vi "WIP_List.vi"(8 "error in (no error)":errorcluster, 10 "Label.Text":string, 11 "Ref in":T1={"MS SQL Connection"=refnum, "UDL File"=path "", "Time"="", "DCODE"="", "WIP+1"=0, "MC No?"=0, "POKAYOKE?"=FALSE, "Expected Result"="", "Result [Status]"="", "Clock"=0.0, "RFID"="", "WIP Queue"=refnum, "TS Parameter"={"ProfitCenterCode"="", "LineCode"="", "WorkOrderNumber"="", "Model"="", "Model_with_Prefix"="", "VendorCode"="", "SetParameterDateCode"="", "PokaYoke"=0, "Target"=1, "Live_DateCode"="", "CustomerPartNumber"="", "Hand"="", "sBarcode"=FALSE, "FCA"=0, "Ent_Stamp"=timestamp(0 s since 1904-01-01), "STS_CD"=0.0}, "Data_Queue"=[], "RFID Serial No."=""} {"TS Parameter"."FCA" format="%01d"; "TS Parameter"."Target" min=1 max=100000; "TS Parameter"."PokaYoke" min=0 max=1}) -> (0 "error out":errorcluster)   [LabVIEW 2020]
uses:
  Controls/TD SQL.ctl
  <vilib>/addons/database/Connection.llb/Conn ObjectReference.ctl
  Controls/WIP_State.ctl
  Controls/TS_Parameter.ctl
  MS SQL/MS_Global.vi
  <vilib>/addons/database/NI_Database_API.lvlib
panel:
  in  "Exit":bool
  in  "WIP List":i32(listbox)
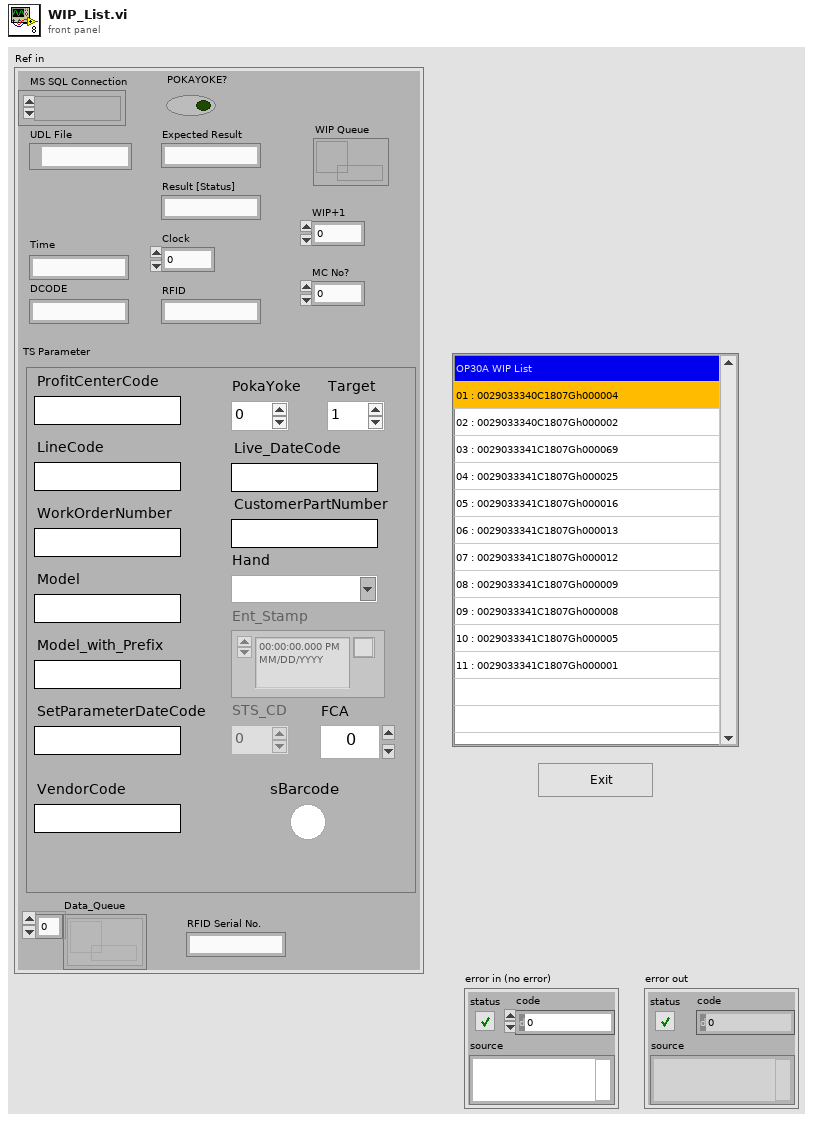
[diagram p1: front panel]
types:
  T1 = typedef "TD SQL.ctl" = cluster{"MS SQL Connection":T2, "UDL File":path, "Time":string, "DCODE":string, "WIP+1":i64, "MC No?":i32, "POKAYOKE?":bool, "Expected Result":string, "Result [Status]":string, "Clock":dbl, "RFID":string, "WIP Queue":refnum<queue>, "TS Parameter":T3, "Data_Queue":refnum<queue>[], "RFID Serial No.":string}
  T2 = typedef "NI_Database_API.lvlib/Conn ObjectReference.ctl" = refnum<k1>
  T3 = typedef "TS_Parameter.ctl" = cluster{"ProfitCenterCode":string, "LineCode":string, "WorkOrderNumber":string, "Model":string, "Model_with_Prefix":string, "VendorCode":string, "SetParameterDateCode":string, "PokaYoke":i32, "Target":i32, "Live_DateCode":string, "CustomerPartNumber":string, "Hand":string, "sBarcode":bool, "FCA":i32, "Ent_Stamp":timestamp, "STS_CD":dbl}
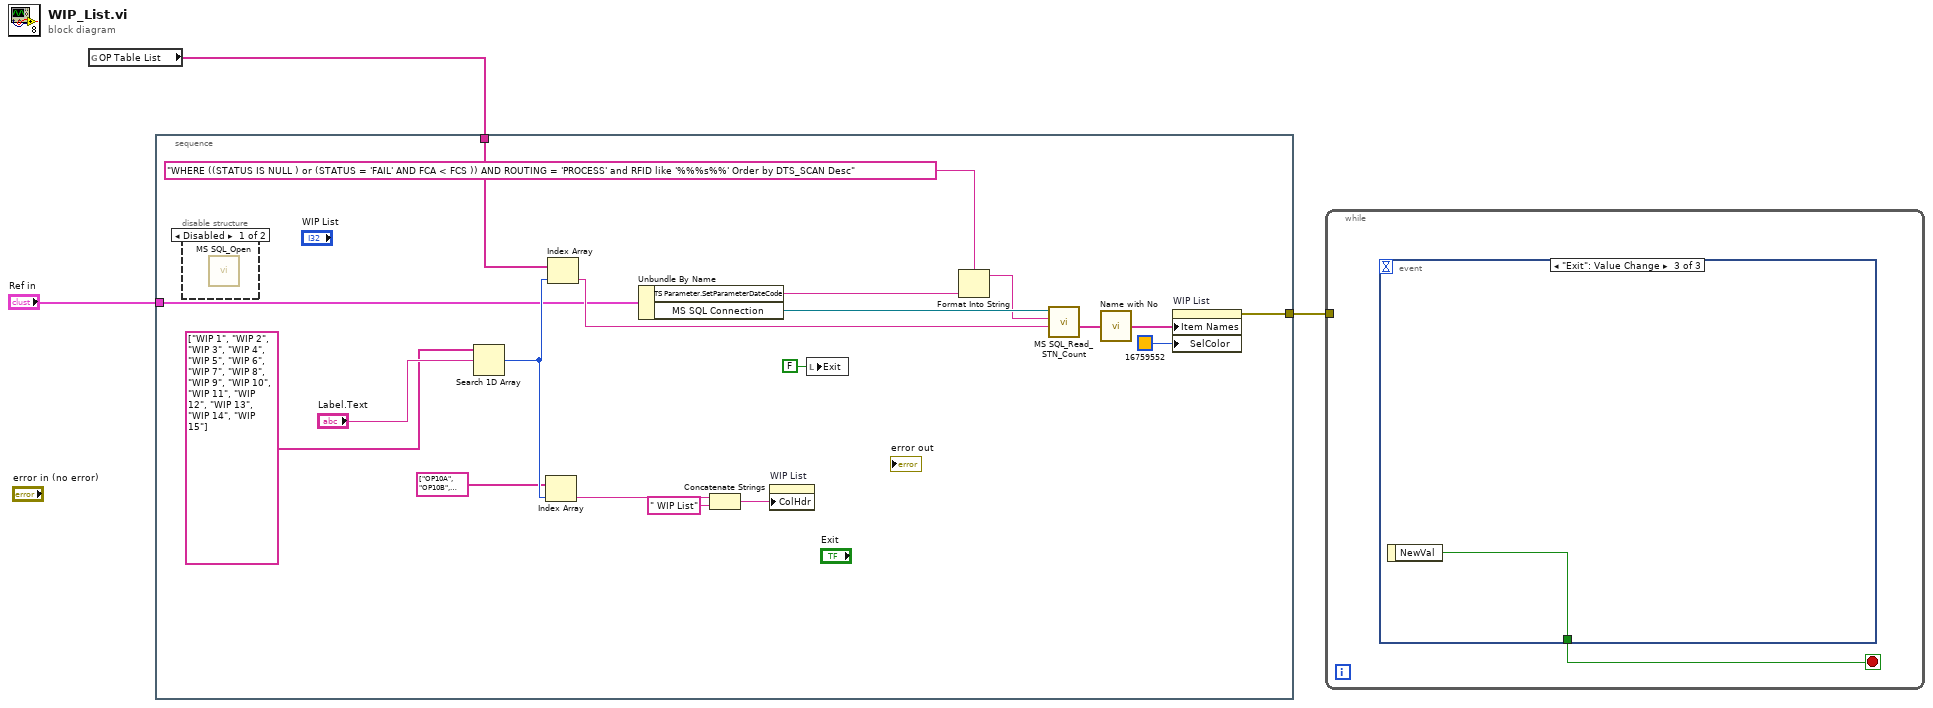
[diagram p0: block diagram]
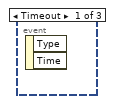
[diagram p3: hidden frame]
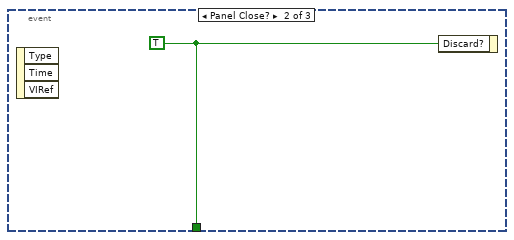
[diagram p4: hidden frame]
diagram:
  n1 = global read "MS_Global.vi" "OP Table List"() -> (w1:string[])
  n2 = stacked-sequence {
    tunnel: "Ref in" -> [w5]
    tunnel: [w16] -> w2
    tunnel: w1 -> [w13]
    frame #0 {
      n3 = disable-structure shown="Disabled" {
        frame Disabled {
          n4 = call "MS SQL_Open.vi"() -> ()  [unwired: 9 in, 3 out]
        }
        frame Enabled {
        }
      }
      n5 = Search 1D Array(1D array=string[] ["WIP 1", "WIP 2", "WIP 3", "WIP 4", "WIP 5", "WIP 6", "WIP 7", "WIP 8", "WIP 9", "WIP 10", "WIP 11", "WIP 12", "WIP 13", "WIP 14", "WIP 15"], element="Label.Text") -> (index of element=w11:i32)  [unwired: 1 in]
      n6 = Index Array(array=string[] ["OP10A", "OP10B", "OP20A", "OP20B", "OP30A", "OP30B", "OP30C", "OP40A", "OP40B", "OP50A", "OP50B", "OP60", "OP70", "OP80"] ("Array"), index=w11) -> (element=w6:string)
      n7 = Index Array(array=w13, index=w11) -> (element=w8:string)
      n8 = Unbundle By Name(w5) -> ("TS Parameter.SetParameterDateCode"=w4:string, "MS SQL Connection"=w20:T2)
      n9 = Concatenate Strings(w6, " WIP List" ("string")) -> (w9:string)
      n10 = property on="WIP List" class="LstBox (strict)"("ColHdr"=w9) -> ()  [unwired: 2 in, 2 out]
      n11 = local write "Exit"(FALSE ("Exit")) -> ()
      n12 = Format Into String(format string="WHERE ((STATUS IS NULL ) or (STATUS = 'FAIL' AND FCA < FCS )) AND ROUTING = 'PROCESS' and RFID like '%%%s%%' Order by DTS_SCAN Desc" ("Query"), w4) -> (resulting string=w18:string)  [unwired: 2 in, 1 out]
      n13 = call "MS SQL_Read_STN_Count.vi"("Table?"=w8, "Query"=w18, "Refnum in"=w20) -> ("RFID"=w14:string[])  [unwired: 5 in, 3 out]
      n14 = call <userlib>:"Name with No.vi"("Seq Name In"=w14) -> ("Seq Name (No.)"=w17:string[])  [unwired: 14 in]
      n15 = property on="WIP List" class="LstBox (strict)"("Item Names"=w17, "SelColor"=u32 16759552 ("Selection Color")) -> (error out=w16:errorcluster)  [unwired: 2 in, 1 out]
    }
  }
  n16 = while {
    tunnel: w2 -> [_]
    stop <- w23 stop-if-true
    n17 = event shown="[2] \"Exit\": Value Change" {
      selector: _ -> [_ _ _]
      dyn-events: _ -> [_ _ _]
      timeout: _ -> [_ _ _]
      tunnel: [_ w24 w25] -> w23
      event Timeout {
        n18 = event-data() -> ()  [unwired: 1 in, 2 out]
      }
      event Panel Close? {
        w24 = TRUE ("Discard?")
        n19 = event-data() -> ()  [unwired: 1 in, 3 out]
        n20 = event-data("Discard?"=w24) -> ()  [unwired: 1 in, 1 out]
      }
      event "Exit": Value Change {
        n21 = event-data() -> ("NewVal"=w25:bool)  [unwired: 1 in]
      }
    }
  }
